vi "Init Task.vi"(4 "counter":tag, 6 "line grouping":i32(ring) items=["one channel for each line", "one channel for all lines"], 7 "physical channels":tag, 8 "error in (no error)":errorcluster, 9 "name":string, 10 "DAQmxTaksContainer_General IN":refnum<class "DAQmxTaksContainer_General.lvclass">, 11 "DAQmxTasklDInput in":refnum<class "DAQmxTaskDInput.lvclass">) -> (0 "error out":errorcluster, 3 "DAQmxTasklDInput out":refnum<class "DAQmxTaskDInput.lvclass">)   [LabVIEW 2019, in "DAQmxTaskDInput.lvclass"]
uses:
  DAQmxTaskDInput.lvclass
  C:/Users/elysium/Documents/dev/TRANCON/Classes/DAQmxTasks/DAQmxTask.lvclass
  DAQmxTaskContainer_General/DAQmxTaksContainer_General.lvclass
  DAQmxTask.lvclass/DAQmxTask.ctl
  <vilib>/DAQmx/create/channels.llb/DAQmx Create Channel (DI-Digital Input).vi
  DAQmxTask.lvclass
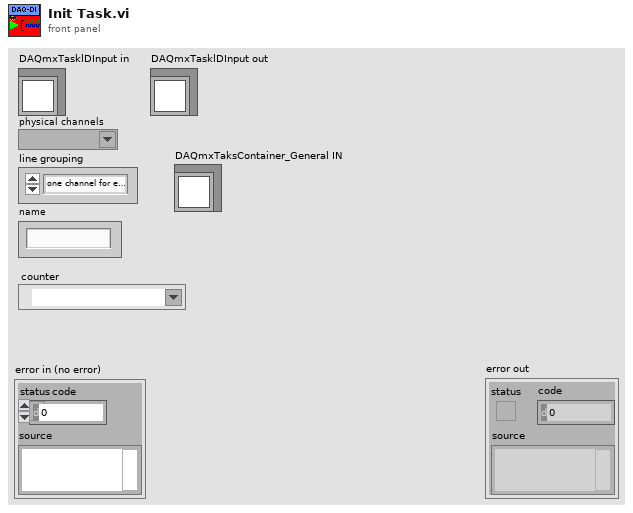
[diagram p1: front panel]
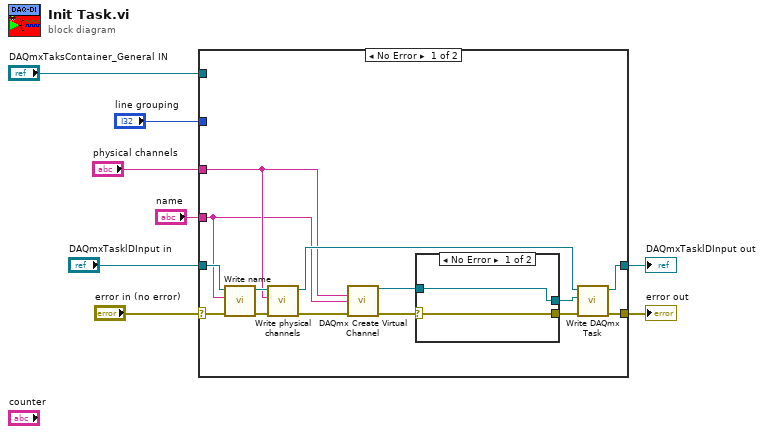
[diagram p0: block diagram]
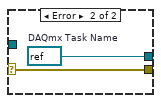
[diagram p2: hidden frame]
diagram:
  n1 = case shown="No Error" "error in (no error)" {
    selector: "error in (no error)" -> [w21 w28]
    tunnel: [w10 w28] -> w7
    tunnel: "DAQmxTasklDInput in" -> [w22 w27]
    tunnel: "name" -> [w11 _]
    tunnel: "physical channels" -> [w17 _]
    tunnel: "line grouping" -> [_ _]
    tunnel: "DAQmxTaksContainer_General IN" -> [_ _]
    tunnel: [w9 w27] -> w1
    frame No Error {
      n2 = call "Write name.vi"("error in (no error)"=w21, "name"=w11, "DAQmxTask in"=w22) -> ("error out"=w19:errorcluster, "DAQmxTask out"=w20:refnum<class "DAQmxTaskDInput.lvclass">)  [unwired: 7 in]
      n3 = call "Write physical channels.vi"("error in (no error)"=w19, "physical channels"=w17, "DAQmxTask in"=w20) -> ("error out"=w12:errorcluster, "DAQmxTask out"=w18:refnum<class "DAQmxTaskDInput.lvclass">)  [unwired: 7 in]
      n4 = call-poly <vilib>:"DAQmx Create Virtual Channel.vi"("lines"=w17, "name to assign"=w11, "error in"=w12) -> ("task out"=w14:refnum<k21>, "error out"=w16:errorcluster)  [unwired: 11 in]
      n5 = case shown="No Error" w16 {
        selector: w16 -> [w23 w25]
        tunnel: [w24 w26] -> w15
        tunnel: w14 -> [w24 _]
        tunnel: [w23 w25] -> w13
        frame No Error {
        }
        frame Error {
          w26 = refnum<k21> refnum  # DAQmx Task Name
        }
      }
      n6 = call "Write DAQmx Task.vi"("error in (no error)"=w13, "DAQmx Task Name"=w15, "DAQmxTask in"=w18) -> ("error out"=w10:errorcluster, "DAQmxTask out"=w9:refnum<class "DAQmxTaskDInput.lvclass">)  [unwired: 7 in]
    }
    frame Error {
    }
  }
  "error out" <- w7
  "DAQmxTasklDInput out" <- w1
